vi "Agilent 681x Acquire Power Measurement.vi"() -> ()   [LabVIEW 2019]
doc: "Shows how to acquire a power measurement using low level data VIs."
uses:
  <vilib>/Utility/error.llb/DialogType.ctl
  <instrlib>/Agilent 681x Series/Public/Data/Low Level/Fetch Single Measurement (Power).vi
  <instrlib>/Agilent 681x Series/Agilent 681x Series.lvlib
panel:
  in  "Sample Spacing (25 us)":dbl=2.5e-05 format="%^.2g"
  in  "Sense Source (0: Internal)":u16(ring) items=["Internal", "External"]
  in  "Output Frequency (60 Hz)":dbl=60.0 format="%#.4g"
  in  "Voltage Amplitude (1.0 V)":dbl=1.0 format="%#.4g"
  in  "Relative Trigger Samples (0)":i32
  in  "Output Waveform Type (0: Sinusoid)":u16(ring) items=["Sinusoid", "Square", "Clipped Sinusoid", "User Specified"]
  out "Total Power":dbl
  out "Power Factor":dbl
  out "Reactive Power":dbl
  out "Apparent Power":dbl
  out "Real Power":dbl
  out "DC Power":dbl
  in  "Maximum Time (10000 ms)":i32=10000
  in  "User-Specified Output Waveform Name":string
  in  "Serial Configuration":T1={"Baud Rate"=9600, "Parity"=0, "Data Bits"=7} {"Data Bits" items=["7"=7, "8"=8]; "Parity" items=["None", "Odd", "Even", "Mark", "Space"]; "Baud Rate" items=["300"=300, "600"=600, "1200"=1200, "2400"=2400, "4800"=4800, "9600"=9600]}
  in  "VISA resource name":refnum<visa-resource-name>
  # "(c) 2008-2021 National Instruments Corp.  ALL RIGHTS RESERVED."
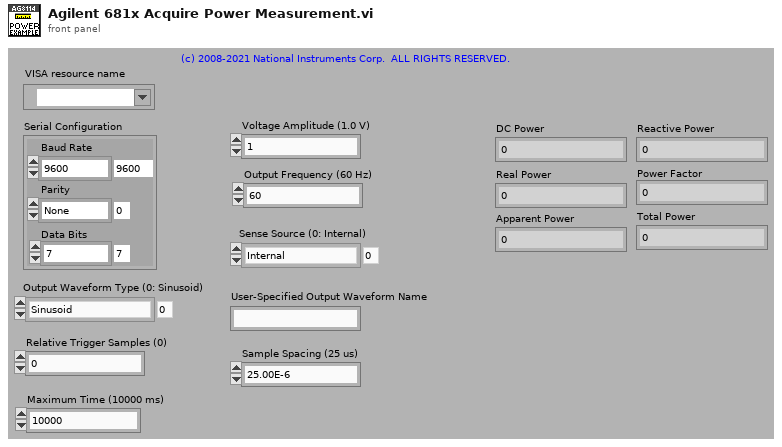
[diagram p1: front panel]
types:
  T1 = cluster{"Baud Rate":u32, "Parity":u16, "Data Bits":u16}
  T2 = typedef "DialogType.ctl" = u16
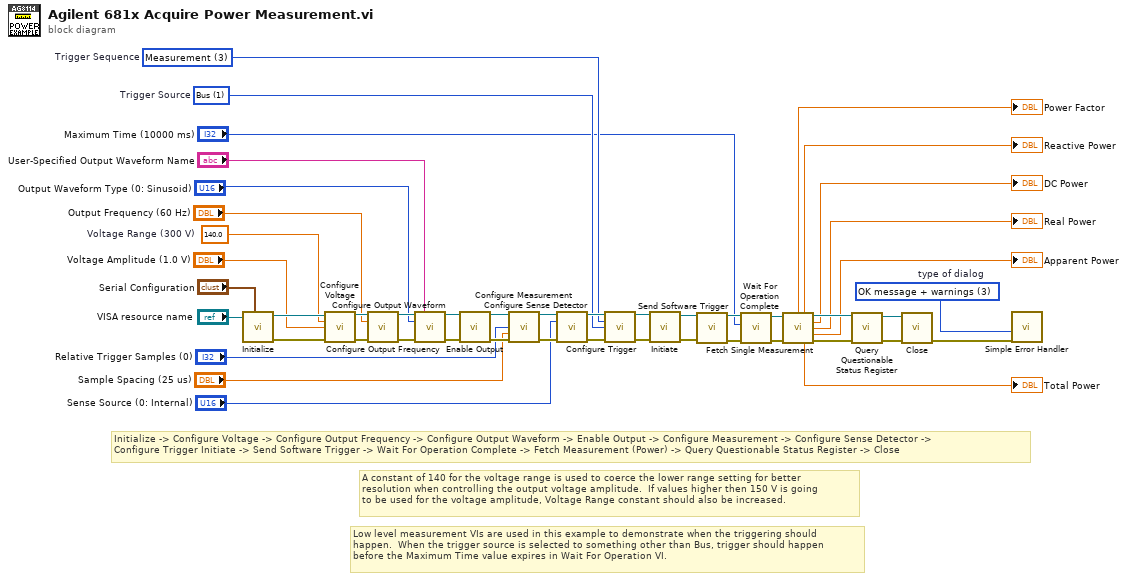
[diagram p0: block diagram]
diagram:
  w8 = T2 3 items=["no dialog", "OK message", "continue or stop message", "OK message + warnings", "continue/stop + warnings"]  # type of dialog
  w28 = 1 items=["Immediate", "Bus", "External", "Phase", "Trigger Out"]  # Trigger Source
  w29 = 3 items=["Output"=1, "Synchronous Source"=2, "Measurement"=3]  # Trigger Sequence
  w43 = 140.0  # Voltage Range (300 V)
  # "Low level measurement VIs are used in this example to demonstrate when the triggering should\nhappen.  When the trigger source is selected to something other than Bus, trigger should happen\nbefore the Maximum Time value expires in Wait For Operation VI."
  # "A constant of 140 for the voltage range is used to coerce the lower range setting for better\nresolution when controlling the output voltage amplitude.  If values higher then 150 V is going\nto be used for the voltage amplitude, Voltage Range constant should also be increased."
  # "Initialize -> Configure Voltage -> Configure Output Frequency -> Configure Output Waveform -> Enable Output -> Configure Measurement -> Configure Sense Detector -> \nConfigure Trigger Initiate -> Send Software Trigger -> Wait For Operation Complete -> Fetch Measurement (Power) -> Query Questionable Status Register -> Close"
  n1 = call <instrlib>:"Initialize.vi"("Serial Configuration"="Serial Configuration", "VISA resource name"="VISA resource name") -> ("error out"=w44:errorcluster, "VISA resource name out"=w45:refnum<visa-resource-name>)  [unwired: 8 in]
  n2 = call <instrlib>:"Configure Voltage.vi"("VISA resource name"=w45, "Voltage Range (300 V)"=w43, "Voltage Amplitude (1.0 V)"="Voltage Amplitude (1.0 V)", "error in (no error)"=w44) -> ("VISA resource name out"=w32:refnum<visa-resource-name>, "error out"=w33:errorcluster)  [unwired: 10 in]
  n3 = call <instrlib>:"Configure Output Frequency.vi"("VISA resource name"=w32, "Output Frequency (60 Hz)"="Output Frequency (60 Hz)", "error in (no error)"=w33) -> ("VISA resource name out"=w39:refnum<visa-resource-name>, "error out"=w40:errorcluster)  [unwired: 11 in]
  n4 = call <instrlib>:"Configure Output Waveform.vi"("VISA resource name"=w39, "User-Specified Output Waveform Name"="User-Specified Output Waveform Name", "Output Waveform Type (0: Sinusoid)"="Output Waveform Type (0: Sinusoid)", "error in (no error)"=w40) -> ("VISA resource name out"=w41:refnum<visa-resource-name>, "error out"=w42:errorcluster)  [unwired: 10 in]
  n5 = call <instrlib>:"Enable Output.vi"("VISA resource name"=w41, "error in (no error)"=w42) -> ("VISA resource name out"=w37:refnum<visa-resource-name>, "error out"=w36:errorcluster)  [unwired: 12 in]
  n6 = call <instrlib>:"Configure Measurement.vi"("VISA resource name"=w37, "Relative Trigger Samples (0)"="Relative Trigger Samples (0)", "Sample Spacing (25 us)"="Sample Spacing (25 us)", "error in (no error)"=w36) -> ("VISA resource name out"=w35:refnum<visa-resource-name>, "error out"=w34:errorcluster)  [unwired: 10 in]
  n7 = call <instrlib>:"Configure Sense Detector.vi"("VISA resource name"=w35, "Sense Source (0: Internal)"="Sense Source (0: Internal)", "error in (no error)"=w34) -> ("VISA resource name out"=w30:refnum<visa-resource-name>, "error out"=w31:errorcluster)  [unwired: 11 in]
  n8 = call <instrlib>:"Configure Trigger.vi"("VISA resource name"=w30, "Trigger Sequence (1: Output 1)"=w29, "Trigger Source (0: Immediate)"=w28, "error in (no error)"=w31) -> ("VISA resource name out"=w26:refnum<visa-resource-name>, "error out"=w27:errorcluster)  [unwired: 10 in]
  n9 = call <instrlib>:"Initiate.vi"("error in (no error)"=w27, "VISA resource name"=w26) -> ("error out"=w24:errorcluster, "VISA resource name out"=w25:refnum<visa-resource-name>)  [unwired: 8 in]
  n10 = call <instrlib>:"Send Software Trigger.vi"("VISA resource name"=w25, "error in (no error)"=w24) -> ("VISA resource name out"=w22:refnum<visa-resource-name>, "error out"=w23:errorcluster)  [unwired: 12 in]
  n11 = call <instrlib>:"Wait For Operation Complete.vi"("error in (no error)"=w23, "Maximum Time (10000 ms)"="Maximum Time (10000 ms)", "VISA resource name"=w22) -> ("error out"=w20:errorcluster, "VISA resource name out"=w21:refnum<visa-resource-name>)  [unwired: 7 in]
  n12 = call-poly <instrlib>:"Fetch Single Measurement.vi"("VISA resource name"=w21, "error in (no error)"=w20) -> ("Power Factor"=→"Power Factor":dbl, "Reactive Power"=→"Reactive Power":dbl, "VISA resource name out"=w18:refnum<visa-resource-name>, "DC Power"=→"DC Power":dbl, "Real Power"=→"Real Power":dbl, "Apparent Power"=→"Apparent Power":dbl, "Total Power"=→"Total Power":dbl, "error out"=w19:errorcluster)  [unwired: 6 in]
  n13 = call <instrlib>:"Query Questionable Status Register.vi"("error in (no error)"=w19, "VISA resource name"=w18) -> ("error out"=w16:errorcluster, "VISA resource name out"=w15:refnum<visa-resource-name>)  [unwired: 7 in, 1 out]
  n14 = call <instrlib>:"Close.vi"("error in (no error)"=w16, "VISA resource name"=w15) -> ("error out"=w17:errorcluster)  [unwired: 9 in]
  n15 = call <vilib>:"Simple Error Handler.vi"("type of dialog (OK msg:1)"=w8, "error in (no error)"=w17) -> ()  [unwired: 3 in, 5 out]
